vi "FPGA Inverse Time Delay (Definite Reset).vi"(0 "pick-up signal? (F)":bool, 1 "number of channels":T2=1 items=["1"=1, "2"=2, "3"=3, "4"=4, "5"=5, "6"=6, "7"=7, "8"=8, "9"=9, "10"=10, "11"=11, "12"=12, "13"=13, "14"=14, "15"=15, "16"=16], 2 "memory info of curve":T1={"reference"="", "size"=240}, 5 "G":fxp<+/-,48,24>, 7 "Gs":fxp<+/-,48,24>, 9 "input valid? (T)":bool=TRUE, 12 "ready for output? (T)":bool=TRUE, 13 "instantaneous reset after tripping? (F)":bool) -> (4 "trip signal?":bool, 10 "output valid?":bool, 14 "ready for input?":bool, 15 "error":i32)   [LabVIEW 2013, in "NI_EP_Protection_FPGA.lvlib"]
doc: "Delays for the time interval that you specify in the Inverse Time Curves VI before the trip signal asserts. The Inverse Time Curves VI generates inverse time curves for this VI to use. You can compensate for the processing delay of the input energizing quantity under a specific G/Gs in the Inverse Time Curves VI to achieve higher operate time accuracy."
uses:
  <vilib>/addons/Electrical Power/Protection/NI_EP_Protection_FPGA.lvlib
  <vilib>/addons/Electrical Power/PQ/Resampling/FPGA/subVIs/fpga_NofCH.ctl
  <vilib>/addons/Electrical Power/Protection/Inverse Time Delay/subVIs/ep_Curve Memory.ctl
  <vilib>/rvi/FXPMathLib/basic elements/FxpDiscreteDelay/XNode/nifxpmath_DiscreteDelay.xnode
  <vilib>/addons/Electrical Power/PQ/Resampling/NI_EP_Resample_FPGA.lvlib
  <vilib>/addons/Electrical Power/Protection/NI_EP_Protection.lvlib
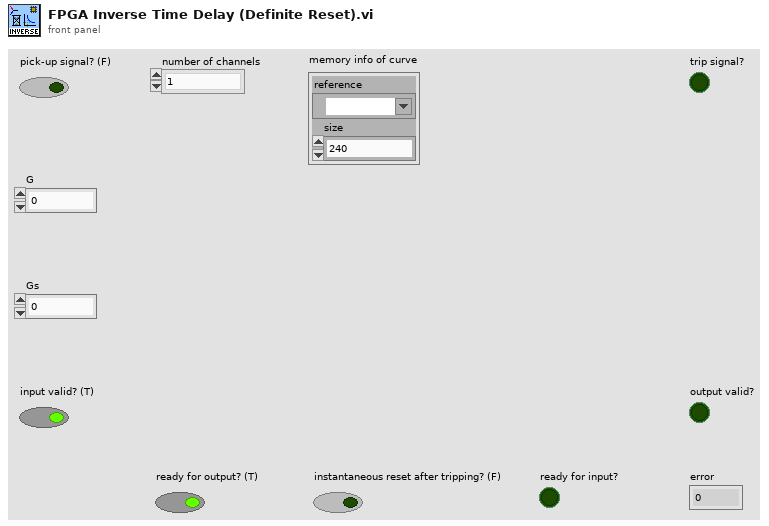
[diagram p1: front panel]
types:
  T1 = typedef "NI_EP_Protection.lvlib/ep_Curve Memory.ctl" = cluster{"reference":refnum<k21>, "size":u16}
  T2 = typedef "NI_EP_Resample_FPGA.lvlib/fpga_NofCH.ctl" = u8
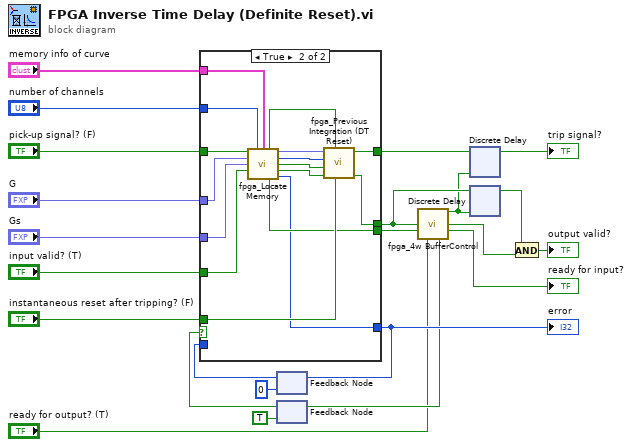
[diagram p0: block diagram]
diagram:
  n1 = feedback #1(0 ("code")) -> (w10:i32)
  n2 = feedback #2(TRUE ("logic enable")) -> (w17:bool)
  n3 = case shown="True" w17 {
    tunnel: "number of channels" -> [_ w33]
    tunnel: [w24 w25] -> w9
    tunnel: "instantaneous reset after tripping? (F)" -> [_ w39]
    tunnel: "memory info of curve" -> [_ w32]
    tunnel: [_ w37] -> w14
    tunnel: "G" -> [_ w30]
    tunnel: "input valid? (T)" -> [_ w28]
    tunnel: "Gs" -> [_ w29]
    tunnel: "pick-up signal? (F)" -> [_ w31]
    tunnel: [_ w35] -> w18
    tunnel: [_ w34] -> w15
    tunnel: w10 -> [w24 _]
    frame False {
    }
    frame True {
      n4 = call <vilib>:"fpga_Locate Memory.vi"("pick-up signal? (F)"=w31, "number of channels"=w33, "memory info of curve"=w32, "G"=w30, "Gs"=w29, "input valid? (T)"=w28) -> ("integrate?"=w27:bool, "dt/T"=w26:fxp<+/-,32,1>, "channel index"=w38:u8, "pick-up signal?"=w36:bool, "output valid"=w40:bool, "ready for input"=w34:bool, "error"=w25:i32)  [unwired: 3 in]
      n5 = call <vilib>:"fpga_Previous Integration (DT Reset).vi"("instantaneous reset after tripping? (F)"=w39, "integrate?"=w27, "input valid"=w40, "start signal? (F)"=w36, "channel index"=w38, "dt/T"=w26) -> ("output valid"=w37:bool, "trip?"=w35:bool)  [unwired: 3 in, 1 out]
    }
  }
  "error" <- w9
  n6 = feedback-in #1(w9) -> ()
  n7 = call <vilib>:"fpga_4w BufferControl.vi"("DR"=w14, "RFI"=w15, "RFO"="ready for output? (T)") -> ("buff enable"=w13:bool, "output valid"=w11:bool, "ready for input"=→"ready for input?":bool, "logic enable"=w7:bool)  [unwired: 9 in]
  n8 = feedback-in #2(w7) -> ()
  n9 = xnode ("Discrete Delay")("D"=w18, "enable"=w13) -> ("Q"=→"trip signal?":bool)
  n10 = xnode ("Discrete Delay")("D"=w14, "enable"=w13) -> ("Q"=w12:bool)
  n11 = And(x=w12, y=w11) -> (x .and. y?=→"output valid?":bool)
